vi "create.ModifyOrderLong.vi"(8 "error in (no error)":errorcluster, 11 "ModifyOrderLong.Parameters":T1={"Time Offset"=447000, "Order Id"="ORID0001", "Quantity"=20000, "Price"=0.905, "Modify Flags"=1}) -> (0 "error out":errorcluster, 2 "Bytes.out":u8[](array[numeric]) format="%.0x", 3 "MessageBase out":refnum<class "ModifyOrderLong.lvclass">)   [LabVIEW 2022 SP3]
uses:
  ModifyOrder/ModifyOrderLong.Parameters.ctl
  ModifyOrder/ModifyOrderLong.lvclass
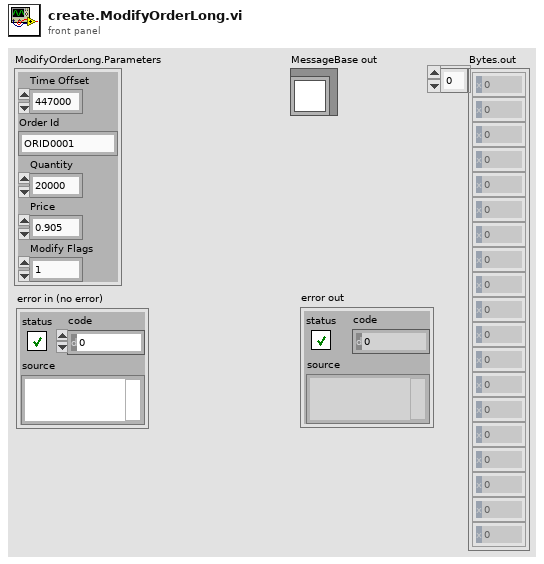
[diagram p1: front panel]
types:
  T1 = typedef "ModifyOrderLong.lvclass/ModifyOrderLong.Parameters.ctl" = cluster{"Time Offset":u32, "Order Id":string, "Quantity":u32, "Price":dbl, "Modify Flags":u8}
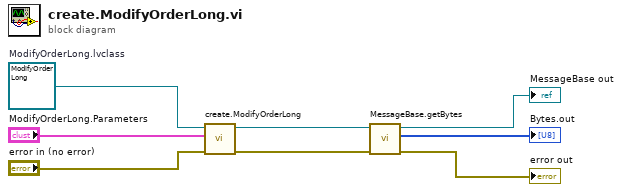
[diagram p0: block diagram]
diagram:
  w6 = refnum<class "ModifyOrderLong.lvclass"> refnum  # ModifyOrderLong.lvclass
  n1 = call-dynamic "create.ModifyOrderLong.vi"("error in"="error in (no error)", "ModifyOrderLong.Parameters"="ModifyOrderLong.Parameters", "ModifyOrderLong in"=w6) -> ("error out"=w1:errorcluster, "ModifyOrderLong out"=w5:refnum<class "ModifyOrderLong.lvclass">)  [unwired: 7 in]
  n2 = call-dynamic "MessageBase.getBytes.vi"("error in (no error)"=w1, "MessageBase in"=w5) -> ("error out"=→"error out":errorcluster, "Bytes.out"=→"Bytes.out":u8[], "MessageBase out"=→"MessageBase out":refnum<class "ModifyOrderLong.lvclass">)  [unwired: 7 in]
